vi "Analysis Info Cluster 2 String.vi"(6 "Analysis Info cluster":T1[](array[typedef]) {"Kurt_u" format="%_3g"; "u^4" format="%_3g"; "u^3" format="%_3g"; "Sd Error in Variance" format="%_3g"; "u^2" format="%_3g"; "Sd Error in Mean" format="%_3g"; "U" format="%_3g"; "Sync Delay Time (s)" format="%.4f"; "Total Meas Time (s)" format="%_5g"; "Skew_u" format="%_3g"; "% u'/U" format="%_3g"}) -> (1 "Output string":string)   [LabVIEW 2022 SP3]
uses:
  Globals/Meas_global.vi
  Controls/Inst_type.ctl
  Controls/Instrument_Array.ctl
  Controls/Analysis_info_cluster.ctl
  Controls/channelState.ctl
panel:
  out "appended array":string[][](array[string])
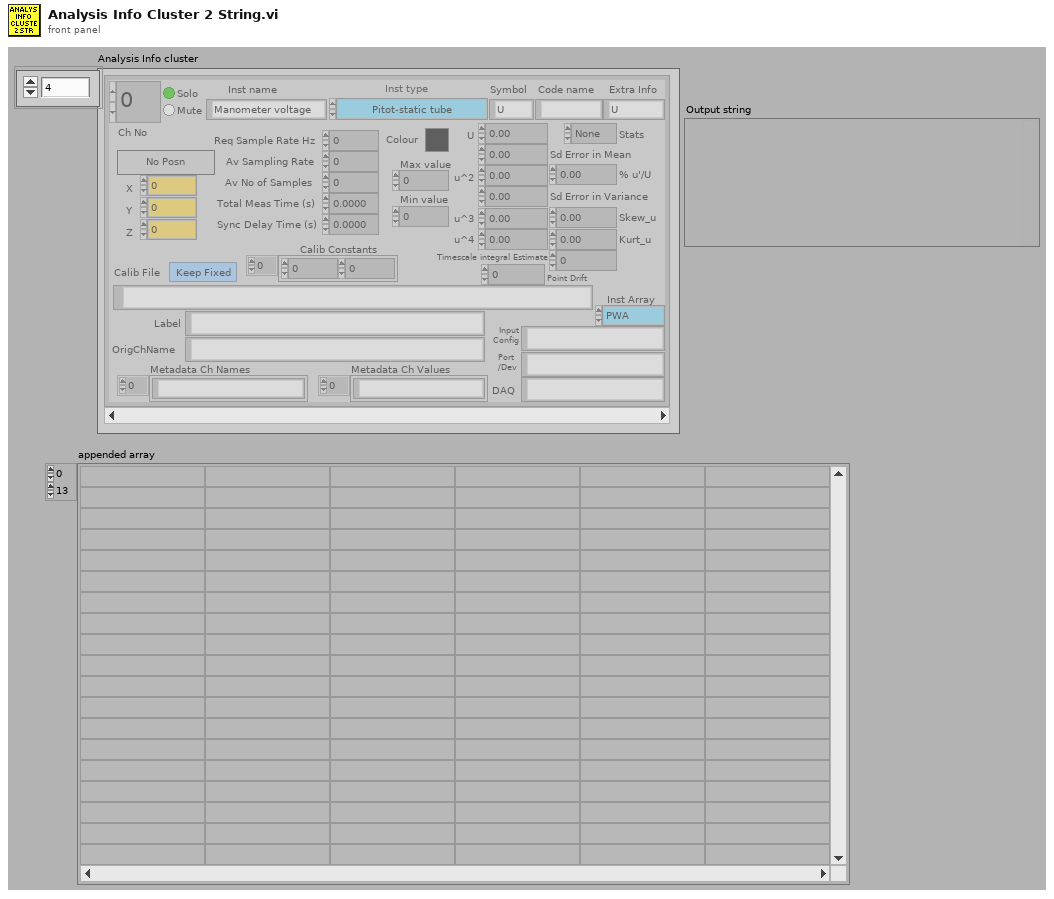
[diagram p1: front panel]
types:
  T1 = typedef "Analysis_info_cluster.ctl" = cluster{"Colour":u32, "Inst type":T2, "Inst name":string, "Symbol":string, "Code name":string, "Extra Info":string, "Inst Array":T3, "U":dbl, "u^2":dbl, "u^3":dbl, "u^4":dbl, "Skew_u":dbl, "Kurt_u":dbl, "Sd Error in Mean":dbl, "% u'/U":dbl, "X":dbl, "Y":dbl, "Z":dbl, "Timescale integral Estimate":dbl, "Sd Error in Variance":dbl, "Calib File":path, "Calib Constants":dbl[], "Output Position":bool, "Stats":enum16{"None", "Basic", "Full"}, "Av Sampling Rate":dbl, "Av No of Samples":dbl, "Total Meas Time (s)":dbl, "OrigChName":string, "Max value":dbl, "Min value":dbl, "Req Sample Rate Hz":dbl, "Sync Delay Time (s)":dbl, "Ch No":i16, "Device":string, "Use Latest Calib":bool, "Port":string, "Metadata Ch Names":string[], "Metadata Ch Values":string[], "Label":string, "chState":T4, "Point Drift":dbl, "inputConfig":string}
  T2 = typedef "Inst_type.ctl" = enum16{"Raw voltage", "Raw with zero offsetting", "Propeller anemometer", "Pressure Transducer", "Pitot-static tube", "Hot wire", "Cross wire 1", "Cross wire 2", "Generic Linear", "Generic Polynomial", "Generic BackPoly", "Fast FID", "Thermocouple", "Cold wire", "Pulsed Wire", "LDA Vel", "LDA Tran time", "LDA Arr time", "Microphone"}
  T3 = typedef "Instrument_Array.ctl" = enum16{"PWA", "LDA", "Analogue"}
  T4 = typedef "channelState.ctl" = enum32{"No Selection", "Solo", "Mute"}
  T5 = typedef "Initial Positions.ctl" = cluster{"Initial XYZ":sgl[], "Traverse Setup":string, "On Axes":string, "Identity String":string}
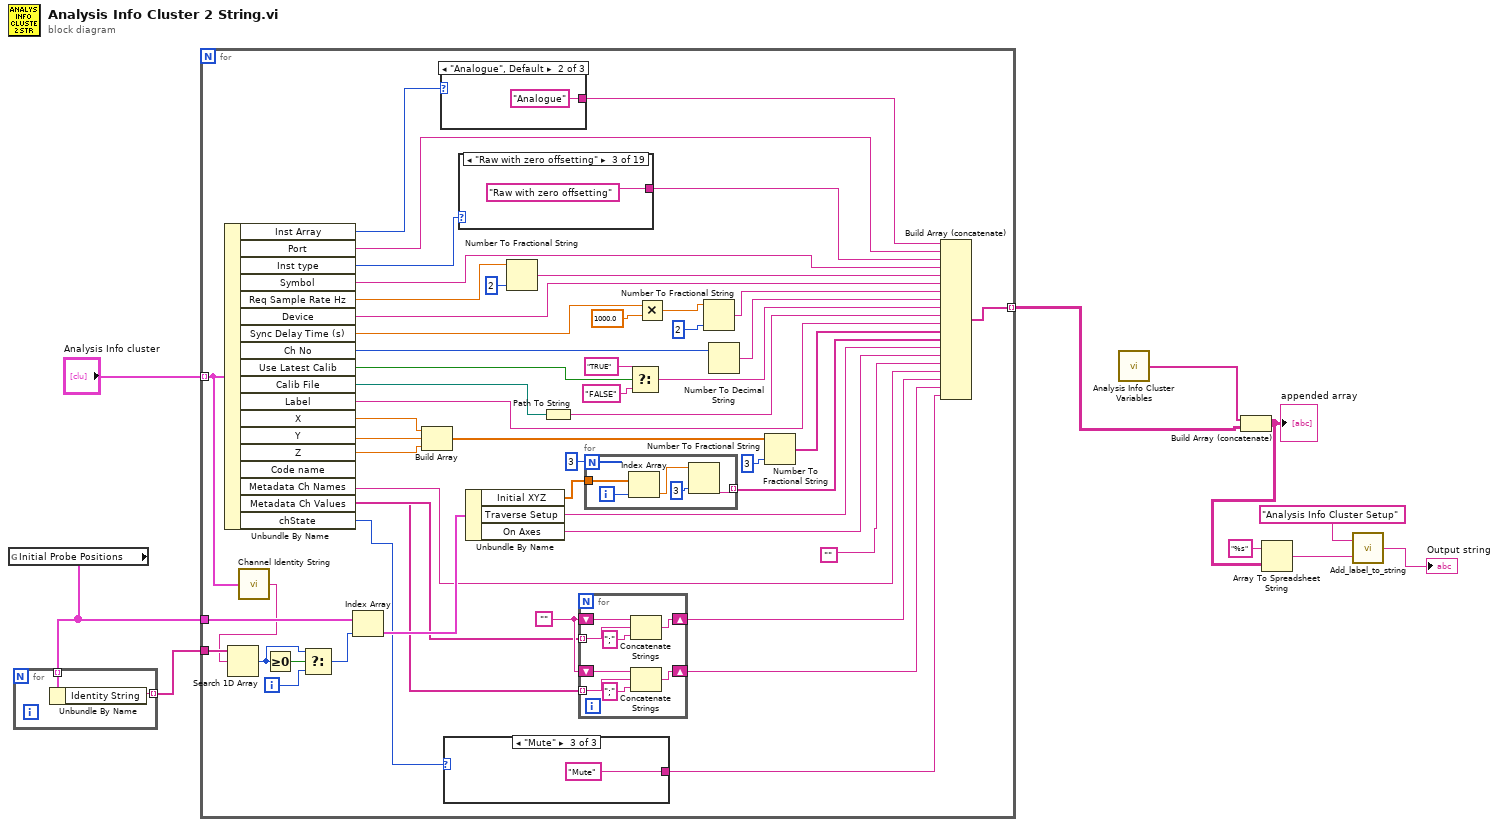
[diagram p0: block diagram]
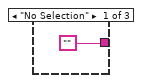
[diagram p2: hidden frame]
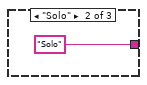
[diagram p3: hidden frame]
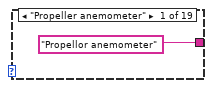
[diagram p4: hidden frame]
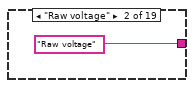
[diagram p5: hidden frame]
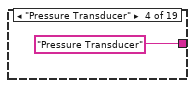
[diagram p6: hidden frame]
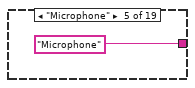
[diagram p7: hidden frame]
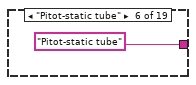
[diagram p8: hidden frame]
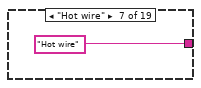
[diagram p9: hidden frame]
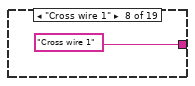
[diagram p10: hidden frame]
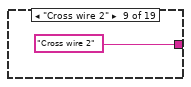
[diagram p11: hidden frame]
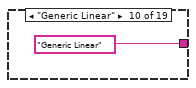
[diagram p12: hidden frame]
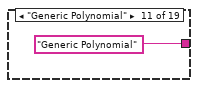
[diagram p13: hidden frame]
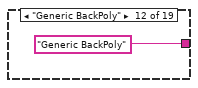
[diagram p14: hidden frame]
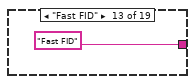
[diagram p15: hidden frame]
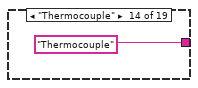
[diagram p16: hidden frame]
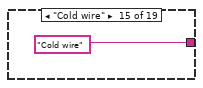
[diagram p17: hidden frame]
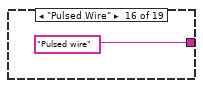
[diagram p18: hidden frame]
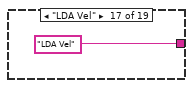
[diagram p19: hidden frame]
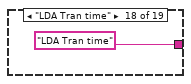
[diagram p20: hidden frame]
diagram:
  n1 = global read "Meas_global.vi" "Initial Probe Positions"() -> (w2:T5[])
  n2 = for {
    tunnel: w2 -> [w12] mode=indexing
    tunnel: [w11] -> w1 mode=indexing
    n3 = Unbundle By Name(w12) -> ("Identity String"=w11:string)
  }
  n4 = for {
    tunnel: "Analysis Info cluster" -> [w23] mode=indexing
    tunnel: [w41] -> w9 mode=indexing
    tunnel: w2 -> [w35]
    tunnel: w1 -> [w25]
    i -> [w19]
    w30 = ""
    n5 = Unbundle By Name(w23) -> ("Inst Array"=w66:T3, "Port"=w64:string, "Inst type"=w63:T2, "Symbol"=w61:string, "Req Sample Rate Hz"=w60:dbl, "Device"=w57:string, "Sync Delay Time (s)"=w55:dbl, "Ch No"=w51:i16, "Use Latest Calib"=w47:bool, "Calib File"=w45:path, "Label"=w36:string, "X"=w38:dbl, "Y"=w39:dbl, "Z"=w40:dbl, "Code name"=w24:string, "Metadata Ch Names"=w29:string[], "Metadata Ch Values"=w28:string[], "chState"=w15:T4)
    n6 = call "Channel Identity String.vi"("Analysis Cluster"=w23) -> ("Identity String"=w21:string)
    n7 = Search 1D Array(1D array=w25, element=w21) -> (index of element=w18:i32)  [unwired: 1 out]
    n8 = Greater Or Equal To 0?(x=w18) -> (x >= 0?=w22:bool)
    n9 = Select(t=w18, s=w22, f=w19) -> (s? t:f=w20:i32)
    n10 = Index Array(array=w35, index=w20) -> (element=w34:T5)
    n11 = Build Array(w38, w39, w40) -> (w42:dbl[])
    n12 = case shown="\"Analogue\", Default" w66 {
      tunnel: ["PWA" "Analogue" "LDA"] -> w65
      frame "PWA" {
      }
      frame "Analogue", Default {
      }
      frame "LDA" {
      }
    }
    n13 = case shown="\"Mute\"" w15 {
      tunnel: ["" "Solo" "Mute"] -> w14
      frame "No Selection" {
      }
      frame "Solo" {
      }
      frame "Mute" {
      }
    }
    n14 = case shown="\"Raw with zero offsetting\"" w63 {
      tunnel: ["Propellor anemometer" "Raw voltage" "Raw with zero offsetting" "Pressure Transducer" "Microphone" "Pitot-static tube" "Hot wire" "Cross wire 1" "Cross wire 2" "Generic Linear" "Generic Polynomial" "Generic BackPoly" "Fast FID" "Thermocouple" "Cold wire" "Pulsed wire" "LDA Vel" "LDA Tran time" "LDA Arr time"] -> w62
      frame "Propeller anemometer" {
      }
      frame "Raw voltage" {
      }
      frame "Raw with zero offsetting" {
      }
      frame "Pressure Transducer" {
      }
      frame "Microphone" {
      }
      frame "Pitot-static tube" {
      }
      frame "Hot wire" {
      }
      frame "Cross wire 1" {
      }
      frame "Cross wire 2" {
      }
      frame "Generic Linear" {
      }
      frame "Generic Polynomial" {
      }
      frame "Generic BackPoly" {
      }
      frame "Fast FID" {
      }
      frame "Thermocouple" {
      }
      frame "Cold wire" {
      }
      frame "Pulsed Wire" {
      }
      frame "LDA Vel" {
      }
      frame "LDA Tran time" {
      }
      frame "LDA Arr time" {
      }
    }
    n15 = Unbundle By Name(w34) -> ("Initial XYZ"=w16:sgl[], "Traverse Setup"=w32:string, "On Axes"=w31:string)
    n16 = Number To Fractional String(number=w60, precision (6)=i16 2) -> (F-format string=w59:string)  [unwired: 2 in]
    n17 = Path To String(path=w45) -> (string=w44:string)
    n18 = for {
      shift-right: [w81] -> w27
      shift-left: w30 -> [w82]
      tunnel: w29 -> [w77] mode=indexing
      shift-right: [w80] -> w26
      shift-left: w30 -> [w78]
      tunnel: w28 -> [w79] mode=indexing
      n19 = Concatenate Strings(w82, w77, ";" ("string")) -> (w81:string)
      n20 = Concatenate Strings(w78, w79, ";" ("string")) -> (w80:string)
    }
    n21 = for {
      N: 3 -> [_]
      tunnel: [w73] -> w33 mode=indexing
      tunnel: w16 -> [w72]
      i -> [w71]
      n22 = Index Array(array=w72, index=w71) -> (element=w70:sgl)
      n23 = Number To Fractional String(number=w70, precision (6)=i16 3) -> (F-format string=w73:string)  [unwired: 2 in]
    }
    n24 = Select(t="TRUE", s=w47, f="FALSE") -> (s? t:f=w46:string)
    n25 = Multiply(x=w55, y=1000.0) -> (x*y=w53:dbl)
    n26 = Number To Fractional String(number=w53, precision (6)=i16 2) -> (F-format string=w52:string)  [unwired: 2 in]
    n27 = Number To Decimal String(number=w51) -> (decimal integer string=w50:string)  [unwired: 1 in]
    n28 = Number To Fractional String(number=w42, precision (6)=i16 3) -> (F-format string=w37:string[])  [unwired: 2 in]
    n29 = Build Array (concatenate)(w65, w64, w62, w61, w59, w57, w52, w50, w46, w44, w36, w37, w33, w32, w31, "", w24, w27, w26, w14) -> (w41:string[])
  }
  n30 = call "Analysis Info Cluster Variables.vi"() -> ("Array"=w8:string[])
  n31 = Build Array (concatenate)(w8, w9) -> (w7:string[][])
  "appended array" <- w7
  n32 = Array To Spreadsheet String(array=w7, 3:"%s" ("format string")) -> (spreadsheet string=w4:string)  [unwired: 1 in]
  n33 = call "Add_label_to_string.vi"("String to write"=w4, "File Label"="Analysis Info Cluster Setup") -> ("Output string"=→"Output string":string)
